vi "GetInputType.vi"(8 "error in (no error)":errorcluster, 10 "inputIndex":i32, 11 "session id in":i32) -> (0 "error out":errorcluster, 2 "InputTypeIndex":i32, 3 "session id out":i32)   [LabVIEW 2017, in "libonnx_wrapper.lvlib"]
doc: "/**\n * @brief Получить код типа данных входного тензора\n * \n * Возвращает числовой код типа элементов тензора согласно спецификации ONNX.\n * Используйте таблицу констант в начале этого файла для расшифровки.\n * \n * @param sessionId [IN] ID сессии\n * @param inputIndex [IN] Индекс входа (0-based)\n * \n * @return int32: Код типа данных (1=FLOAT32, 2=FLOAT64, 5=INT32, 6=INT64, ...)\n * @return int32: -1 если сессия не найдена или индекс неверен\n * \n * @see GetInputTypeString для получения читаемого имени типа\n */\nint GetInputType(int sessionId, int inputIndex);"
uses:
  libonnx_wrapper.lvlib
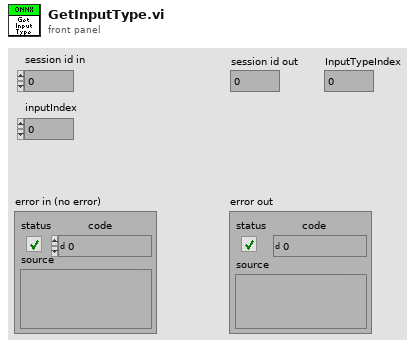
[diagram p1: front panel]
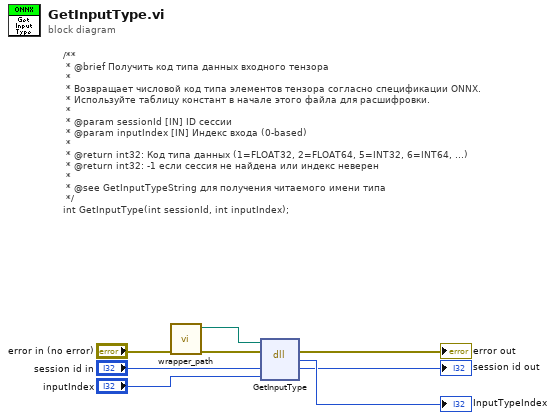
[diagram p0: block diagram]
diagram:
  # "/**\n * @brief Получить код типа данных входного тензора\n * \n * Возвращает числовой код типа элементов тензора согласно спецификации ONNX.\n * Используйте таблицу констант в начале этого файла для расшифровки.\n * \n * @param sessionId [IN] ID сессии\n * @param inputIndex [IN] Индекс входа (0-based)\n * \n * @return int32: Код типа данных (1=FLOAT32, 2=FLOAT64, 5=INT32, 6=INT64, ...)\n * @return int32: -1 если сессия не найдена или индекс неверен\n * \n * @see GetInputTypeString для получения читаемого имени типа\n */\nint GetInputType(int sessionId, int inputIndex);"
  n1 = call "wrapper_path.vi"("error in (no error)"="error in (no error)") -> ("error out"=w2:errorcluster, "wrapper path"=w5:path)  [unwired: 9 in]
  n2 = dll-call lib="home/ivan/LabVIEWData/ONNX/Test/libonnx_wrapper/unix64/libonnx_wrapper.so" fn="GetInputType"(path in=w5, error in=w2, "sessionId"="session id in", "inputIndex"="inputIndex") -> (error out=→"error out":errorcluster, "InputTypeIndex"=→"InputTypeIndex":i32, "sessionId"=→"session id out":i32)  [unwired: 2 in, 1 out]
